vi "Get Shooting Values.vi"() -> ()   [LabVIEW 2020]
uses:
  ae667ebd-e1a2-4ae9-a299-bd2dfb6ddb01.vi
panel:
  out "high flywheel":dbl
  out "low flywheel":dbl
  in  "distance":dbl
  in  "degree":u16=4
  in  "Shooting Table":dbl[][](array[numeric])
  # "Distance, low, high"
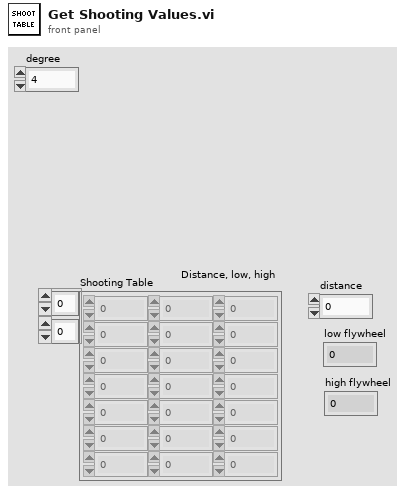
[diagram p1: front panel]
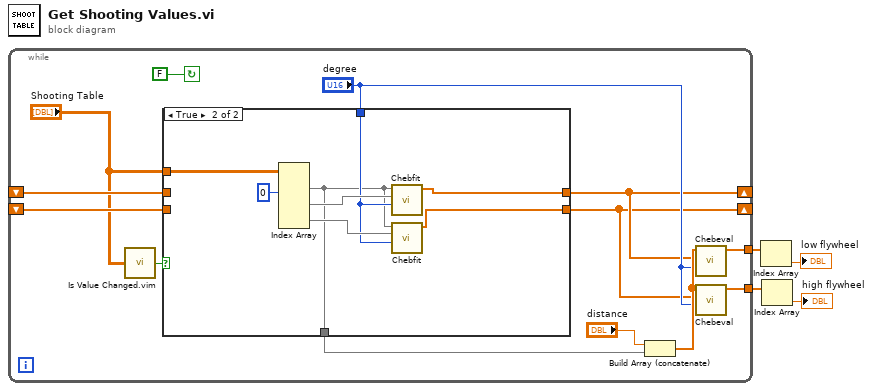
[diagram p0: block diagram]
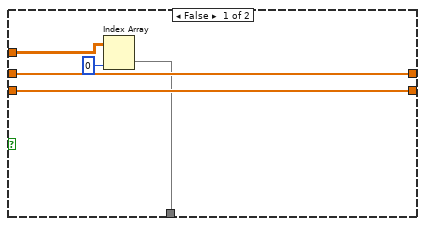
[diagram p2: hidden frame]
diagram:
  n1 = while {
    tunnel: [w14] -> w4
    tunnel: [w13] -> w3
    shift-right: [w12] -> _
    shift-left: _ -> [w10]
    shift-right: [w11] -> _
    shift-left: _ -> [w9]
    stop <- FALSE continue-if-true
    n2 = call "Is Value Changed.vim"("value"="Shooting Table") -> ("changed or first call?"=w7:bool)
    n3 = case shown="True" w7 {
      tunnel: "degree" -> [_ w27]
      tunnel: [w22 w26] -> w12
      tunnel: [w21 w25] -> w11
      tunnel: w10 -> [w22 _]
      tunnel: w9 -> [w21 _]
      tunnel: "Shooting Table" -> [w20 w24]
      tunnel: [w18 w23] -> w5
      frame False {
        n4 = Index Array(array=w20, index (col)=0 ("disabled index (col)")) -> (element=w18:dbl[])  [unwired: 1 in]
      }
      frame True {
        n5 = Index Array(array=w24, index (col) #1=0 ("disabled index (col)")) -> (element #1=w23:dbl[], element #2=w29:dbl[], element #3=w28:dbl[])  [unwired: 5 in]
        n6 = call "Chebfit.vi"("degree"=w27, "Y"=w29, "X"=w23) -> ("C"=w26:dbl[])  [unwired: 8 in]
        n7 = call "Chebfit.vi"("degree"=w27, "Y"=w28, "X"=w23) -> ("C"=w25:dbl[])  [unwired: 8 in]
      }
    }
    n8 = Build Array (concatenate)("distance", w5) -> (w16:dbl[])
    n9 = call "Chebeval.vi"("degree"="degree", "Cheby weights"=w12, "x"=w16) -> ("y"=w14:dbl[])  [unwired: 8 in]
    n10 = call "Chebeval.vi"("degree"="degree", "Cheby weights"=w11, "x"=w16) -> ("y"=w13:dbl[])  [unwired: 8 in]
  }
  n11 = Index Array(array=w4) -> (element=→"low flywheel":dbl)  [unwired: 1 in]
  n12 = Index Array(array=w3) -> (element=→"high flywheel":dbl)  [unwired: 1 in]
